vi "Lichen Analysis2.vi"(0 "Parameters (Rejilla)":T2(array[cluster])=[{"Name"="Rectangle 1", "Type"=enum."Rotated Rectangle", "Coordinates"=[0, 0, 80, 76, 0], "Colors"=[16711680], "Drawing Mode"=0, "Text"="Your Text", "Results"=[], "Font, Size & Style"={"Desired Font (Application)"=enum."System Font", "[User-specified Font]"={"Font Name"="Tahoma", "Size"=13, "Strikeout?"=FALSE, "Italic?"=FALSE, "Underline?"=FALSE, "Outline?"=FALSE, "Shadow?"=FALSE, "Bold?"=FALSE, "Rotation Angle"=0.0}, "Horizontal Alignment"=0, "Vertical Alignment"=0}, "Image File Path"=path "", "Use Keying Color"=FALSE}, {"Name"="Rectangle 2", "Type"=enum."Rotated Rectangle", "Coordinates"=[81, 0, 161, 76, 0], "Colors"=[16717824], "Drawing Mode"=0, "Text"="Your Text", "Results"=[], "Font, Size & Style"={"Desired Font (Application)"=enum."System Font", "[User-specified Font]"={"Font Name"="Tahoma", "Size"=13, "Strikeout?"=FALSE, "Italic?"=FALSE, "Underline?"=FALSE, "Outline?"=FALSE, "Shadow?"=FALSE, "Bold?"=FALSE, "Rotation Angle"=0.0}, "Horizontal Alignment"=0, "Vertical Alignment"=0}, "Image File Path"=path "", "Use Keying Color"=FALSE}, {"Name"="Rectangle 3", "Type"=enum."Rotated Rectangle", "Coordinates"=[0, 77, 80, 152, 0], "Colors"=[16717824], "Drawing Mode"=0, "Text"="Your Text", "Results"=[], "Font, Size & Style"={"Desired Font (Application)"=enum."System Font", "[User-specified Font]"={"Font Name"="Tahoma", "Size"=13, "Strikeout?"=FALSE, "Italic?"=FALSE, "Underline?"=FALSE, "Outline?"=FALSE, "Shadow?"=FALSE, "Bold?"=FALSE, "Rotation Angle"=0.0}, "Horizontal Alignment"=0, "Vertical Alignment"=0}, "Image File Path"=path "", "Use Keying Color"=FALSE}, {"Name"="Rectangle 4", "Type"=enum."Rotated Rectangle", "Coordinates"=[81, 77, 161, 152, 0], "Colors"=[16717824], "Drawing Mode"=0, "Text"="Your Text", "Results"=[], "Font, Size & Style"={"Desired Font (Application)"=enum."System Font", "[User-specified Font]"={"Font Name"="Tahoma", "Size"=13, "Strikeout?"=FALSE, "Italic?"=FALSE, "Underline?"=FALSE, "Outline?"=FALSE, "Shadow?"=FALSE, "Bold?"=FALSE, "Rotation Angle"=0.0}, "Horizontal Alignment"=0, "Vertical Alignment"=0}, "Image File Path"=path "", "Use Keying Color"=FALSE}, {"Name"="Rectangle 5", "Type"=enum."Rotated Rectangle", "Coordinates"=[0, 153, 80, 228, 0], "Colors"=[16717824], "Drawing Mode"=0, "Text"="Your Text", "Results"=[], "Font, Size & Style"={"Desired Font (Application)"=enum."System Font", "[User-specified Font]"={"Font Name"="Tahoma", "Size"=13, "Strikeout?"=FALSE, "Italic?"=FALSE, "Underline?"=FALSE, "Outline?"=FALSE, "Shadow?"=FALSE, "Bold?"=FALSE, "Rotation Angle"=0.0}, "Horizontal Alignment"=0, "Vertical Alignment"=0}, "Image File Path"=path "", "Use Keying Color"=FALSE}, {"Name"="Rectangle 6", "Type"=enum."Rotated Rectangle", "Coordinates"=[81, 153, 161, 228, 0], "Colors"=[16717824], "Drawing Mode"=0, "Text"="Your Text", "Results"=[], "Font, Size & Style"={"Desired Font (Application)"=enum."System Font", "[User-specified Font]"={"Font Name"="Tahoma", "Size"=13, "Strikeout?"=FALSE, "Italic?"=FALSE, "Underline?"=FALSE, "Outline?"=FALSE, "Shadow?"=FALSE, "Bold?"=FALSE, "Rotation Angle"=0.0}, "Horizontal Alignment"=0, "Vertical Alignment"=0}, "Image File Path"=path "", "Use Keying Color"=FALSE}, {"Name"="Text 1", "Type"=enum."Text", "Coordinates"=[3, 73], "Colors"=[2817810, 16777216], "Drawing Mode"=0, "Text"="Cell 1", "Results"=[], "Font, Size & Style"={"Desired Font (Application)"=enum."System Font", "[User-specified Font]"={"Font Name"="Tahoma", "Size"=13, "Strikeout?"=FALSE, "Italic?"=FALSE, "Underline?"=FALSE, "Outline?"=FALSE, "Shadow?"=FALSE, "Bold?"=FALSE, "Rotation Angle"=0.0}, "Horizontal Alignment"=0, "Vertical Alignment"=0}, "Image File Path"=path "", "Use Keying Color"=FALSE}, {"Name"="Text 2", "Type"=enum."Text", "Coordinates"=[83, 73], "Colors"=[2817810, 16777216], "Drawing Mode"=0, "Text"="Cell 2", "Results"=[], "Font, Size & Style"={"Desired Font (Application)"=enum."System Font", "[User-specified Font]"={"Font Name"="Tahoma", "Size"=13, "Strikeout?"=FALSE, "Italic?"=FALSE, "Underline?"=FALSE, "Outline?"=FALSE, "Shadow?"=FALSE, "Bold?"=FALSE, "Rotation Angle"=0.0}, "Horizontal Alignment"=0, "Vertical Alignment"=0}, "Image File Path"=path "", "Use Keying Color"=FALSE}, {"Name"="Text 3", "Type"=enum."Text", "Coordinates"=[3, 149], "Colors"=[2817810, 16777216], "Drawing Mode"=0, "Text"="Cell 3", "Results"=[], "Font, Size & Style"={"Desired Font (Application)"=enum."System Font", "[User-specified Font]"={"Font Name"="Tahoma", "Size"=13, "Strikeout?"=FALSE, "Italic?"=FALSE, "Underline?"=FALSE, "Outline?"=FALSE, "Shadow?"=FALSE, "Bold?"=FALSE, "Rotation Angle"=0.0}, "Horizontal Alignment"=0, "Vertical Alignment"=0}, "Image File Path"=path "", "Use Keying Color"=FALSE}, {"Name"="Text 4", "Type"=enum."Text", "Coordinates"=[83, 149], "Colors"=[2817810, 16777216], "Drawing Mode"=0, "Text"="Cell 4", "Results"=[], "Font, Size & Style"={"Desired Font (Application)"=enum."System Font", "[User-specified Font]"={"Font Name"="Tahoma", "Size"=13, "Strikeout?"=FALSE, "Italic?"=FALSE, "Underline?"=FALSE, "Outline?"=FALSE, "Shadow?"=FALSE, "Bold?"=FALSE, "Rotation Angle"=0.0}, "Horizontal Alignment"=0, "Vertical Alignment"=0}, "Image File Path"=path "", "Use Keying Color"=FALSE}, {"Name"="Text 5", "Type"=enum."Text", "Coordinates"=[3, 225], "Colors"=[2817810, 16777216], "Drawing Mode"=0, "Text"="Cell 5", "Results"=[], "Font, Size & Style"={"Desired Font (Application)"=enum."System Font", "[User-specified Font]"={"Font Name"="Tahoma", "Size"=13, "Strikeout?"=FALSE, "Italic?"=FALSE, "Underline?"=FALSE, "Outline?"=FALSE, "Shadow?"=FALSE, "Bold?"=FALSE, "Rotation Angle"=0.0}, "Horizontal Alignment"=0, "Vertical Alignment"=0}, "Image File Path"=path "", "Use Keying Color"=FALSE}, {"Name"="Text 6", "Type"=enum."Text", "Coordinates"=[83, 225], "Colors"=[65407, 16777216], "Drawing Mode"=0, "Text"="Cell 6", "Results"=[], "Font, Size & Style"={"Desired Font (Application)"=enum."System Font", "[User-specified Font]"={"Font Name"="Tahoma", "Size"=13, "Strikeout?"=FALSE, "Italic?"=FALSE, "Underline?"=FALSE, "Outline?"=FALSE, "Shadow?"=FALSE, "Bold?"=FALSE, "Rotation Angle"=0.0}, "Horizontal Alignment"=0, "Vertical Alignment"=0}, "Image File Path"=path "", "Use Keying Color"=FALSE}] {"Colors" format="%.0x"; "Drawing Mode" items=["Frame", "Fill", "Highlight"]; "Results"."String Format" items=["Decimal", "Hexadecimal", "Octal", "Fractional", "Exponential", "Engineering"]; "Font, Size & Style"."Horizontal Alignment" items=["Left", "Center", "Right"]; "Font, Size & Style"."Vertical Alignment" items=["Bottom", "Top", "Baseline"]}, 7 "error in":errorcluster) -> ()   [LabVIEW 2018]
uses:
  <vilib>/vision/NI_Vision_Development_Module.lvlib
panel:
  in  "StationId":u32=1
  out "Array 2":bool[][](array[boolean])
  out "Array":bool[](array[boolean])
  in  "Rows (Default: 3)":i32=3
  in  "Cols (Default: 2)":i32=2
  out "Lichens":T1[](array[plugin-control])
  out "Pixeles":i32[](array[numeric])
  out "?":sgl[](array[numeric])
  out "Original":T1(plugin-control)
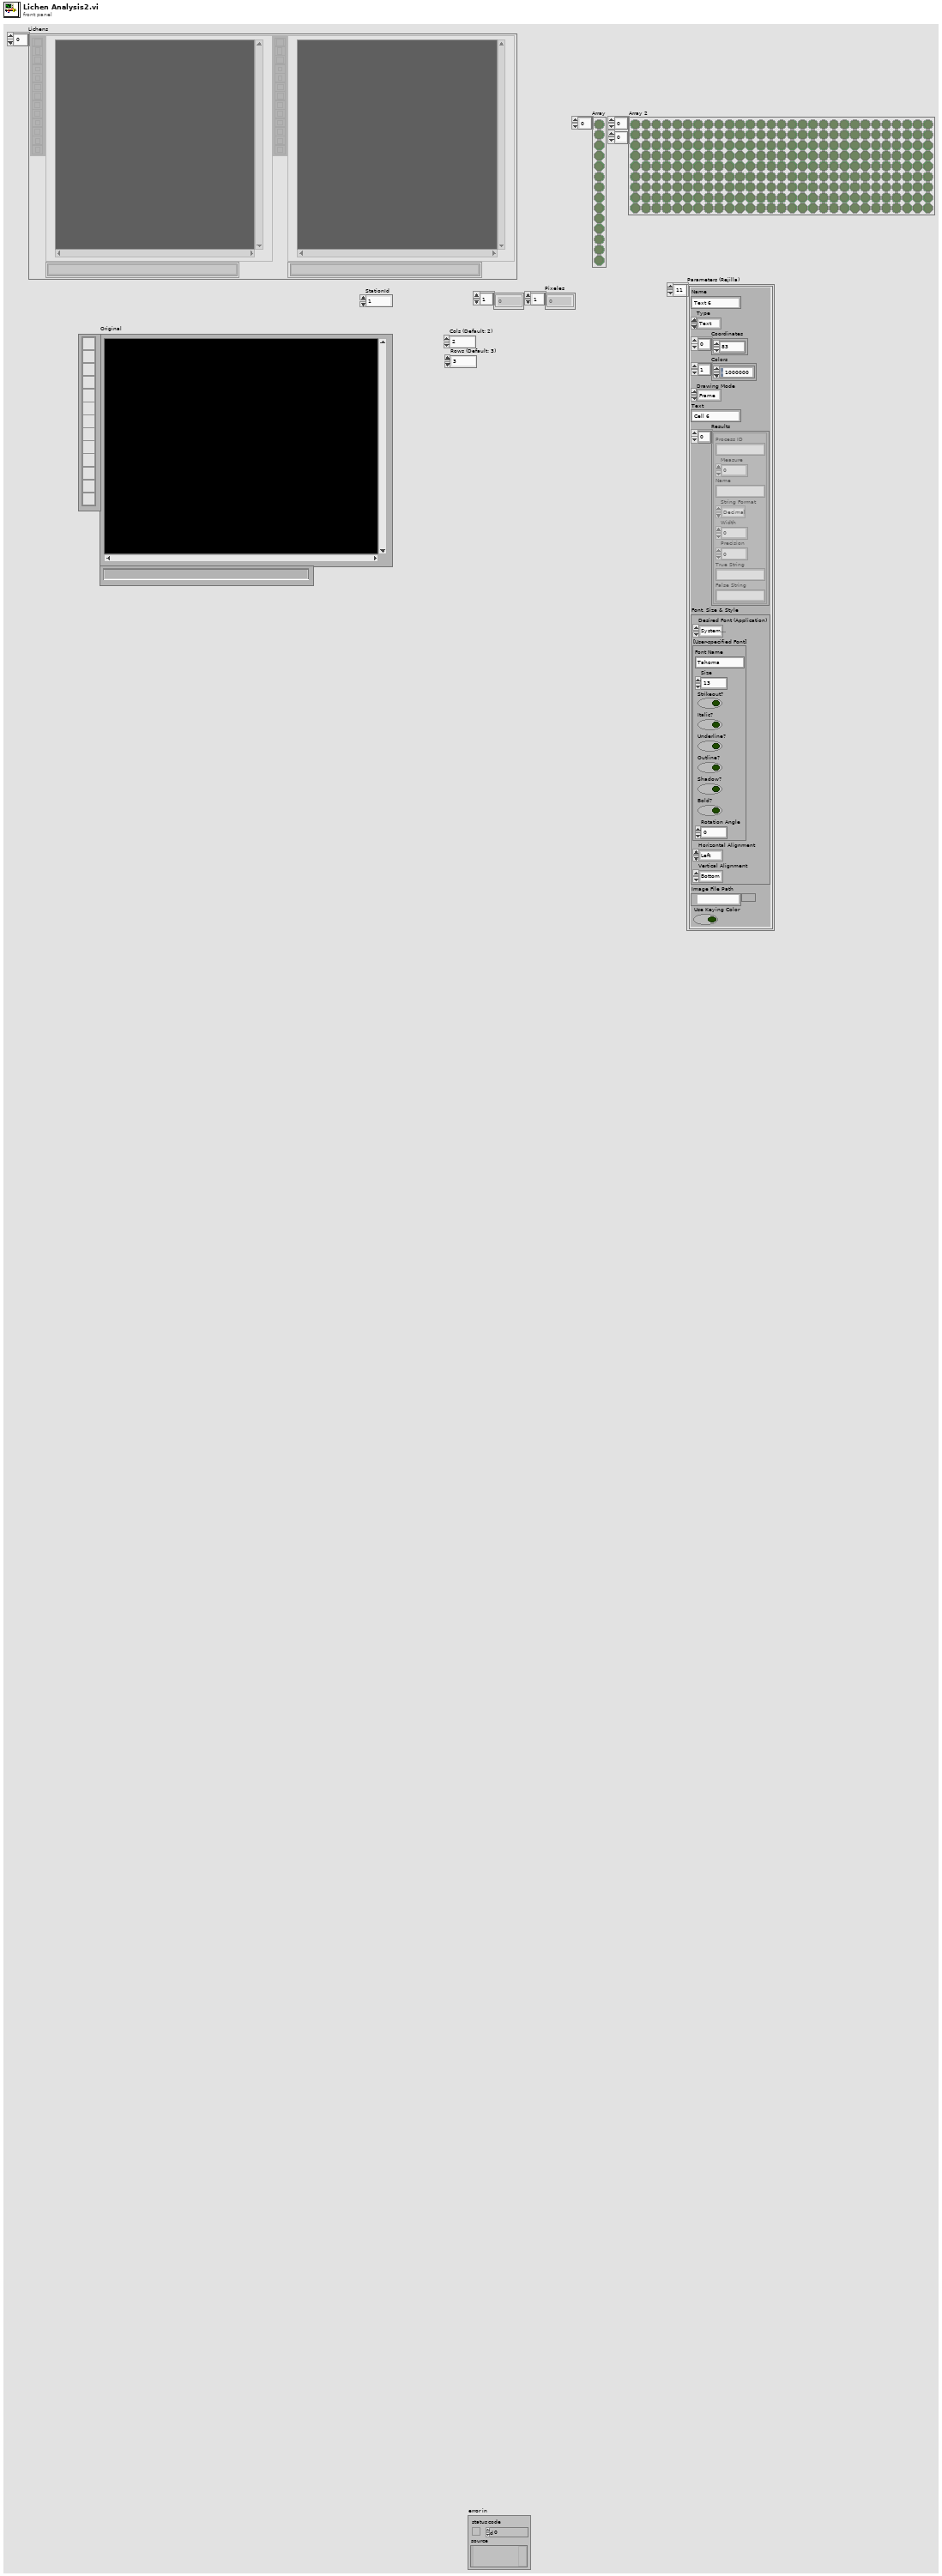
[diagram p1: front panel]
types:
  T1 = typedef "IMAQ Image.ctl" = refnum<image>
  T2 = cluster{"Name":string, "Type":enum16{"Line", "Broken Line", "Free Hand Line", "Rotated Rectangle", "Oval", "Polygon", "Free Hand", "Bitmap", "Text"}, "Coordinates":i32[], "Colors":u32[], "Drawing Mode":u32, "Text":string, "Results":cluster{"Process ID":string, "Measure":u16, "Name":string, "String Format":u16, "Width":i16, "Precision":i16, "True String":string, "False String":string}[], "Font, Size & Style":cluster{"Desired Font (Application)":enum16{"User-specified Font", "Application Font", "System Font", "Dialog Font"}, "[User-specified Font]":cluster{"Font Name":string, "Size":i16, "Strikeout?":bool, "Italic?":bool, "Underline?":bool, "Outline?":bool, "Shadow?":bool, "Bold?":bool, "Rotation Angle":dbl}, "Horizontal Alignment":i16, "Vertical Alignment":i16}, "Image File Path":path, "Use Keying Color":bool}[]
  T3 = typedef "Image Type" = u32
  T4 = cluster{"Position":cluster{"x":sgl, "y":sgl}, "Angle":sgl, "Scale":sgl, "Score":sgl, "Bounding Box":cluster{"x":sgl, "y":sgl}[]}[]
  T5 = cluster{"histogram":u32[], "Minimal Value":sgl, "Maximal Value":sgl, "Starting Value":sgl, "Interval Width":sgl, "Mean Value":sgl, "Standard  Variation":sgl, "Area (pixels)":i32}
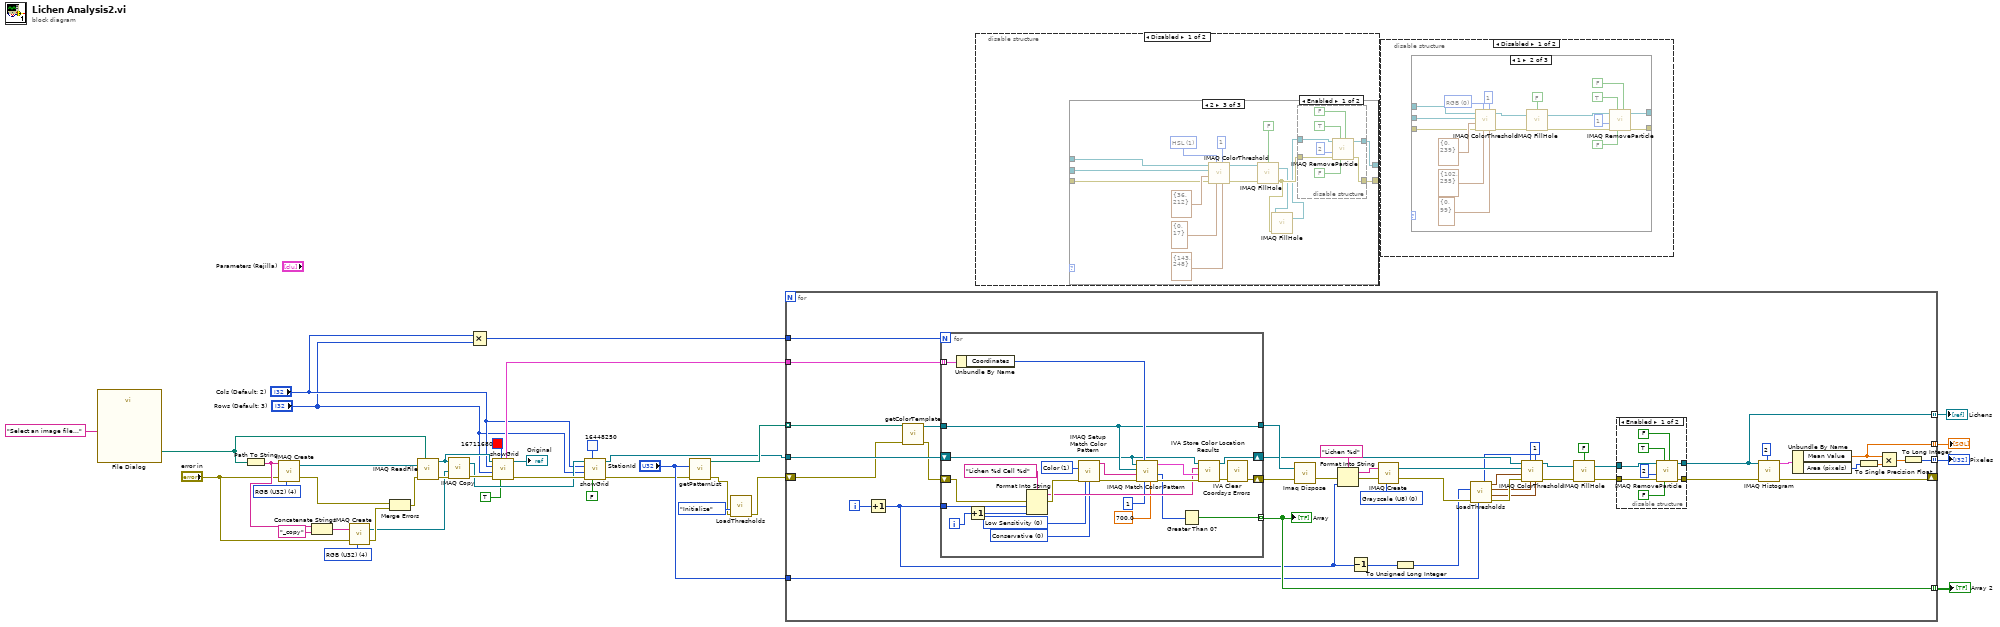
[diagram p0: block diagram]
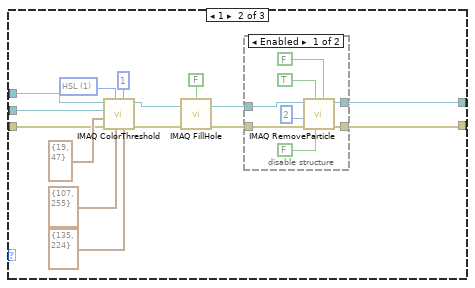
[diagram p3: hidden frame]
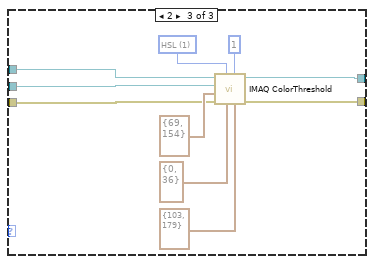
[diagram p8: hidden frame]
diagram:
  w14 = T3 4 items=["Grayscale (U8)", "Grayscale (I16)", "Grayscale (SGL)", "Complex (CSG)", "RGB (U32)", "HSL (U32)", "RGB (U64)", "Grayscale (U16)"] ("Image Type")
  w37 = T3 4 items=["Grayscale (U8)", "Grayscale (I16)", "Grayscale (SGL)", "Complex (CSG)", "RGB (U32)", "HSL (U32)", "RGB (U64)", "Grayscale (U16)"] ("Image Type")
  n1 = call "File Dialog"("prompt"="Select an image file...") -> ("selected path"=w35:path)  [unwired: 6 in, 8 out]
  n2 = Path To String(path=w35) -> (string=w20:string)
  n3 = call "IMAQ Create"("Image Name"=w20, "Image Type"=w37, "error in (no error)"="error in") -> ("New Image"=w36:T1, "error out"=w15:errorcluster)  [unwired: 1 in, 1 out]
  n4 = Concatenate Strings(w20, "_copy" ("string")) -> (w18:string)
  n5 = call "IMAQ Create"("Image Name"=w18, "Image Type"=w14, "error in (no error)"="error in") -> ("New Image"=w12:T1, "error out"=w16:errorcluster)  [unwired: 1 in, 1 out]
  n6 = Merge Errors(w15, w16) -> (w13:errorcluster)
  n7 = call "IMAQ ReadFile"("File Path"=w35, "error in (no error)"=w13, "Image"=w36) -> ("error out"=w22:errorcluster, "Image Out"=w11:T1)  [unwired: 2 in, 5 out]
  n8 = call "IMAQ Copy"("error in (no error)"=w22, "Image Dst"=w12, "Image Src"=w11) -> ("error out"=w21:errorcluster, "Image Dst Out"=w8:T1)  [unwired: 3 in]
  n9 = Multiply(x="Cols (Default: 2)", y="Rows (Default: 3)") -> (x*y=w27:i32)
  n10 = call "showGrid.vi"("Append Text? (True)"=TRUE, "Color (Red)"=u32 16711680, "error in (no error)"=w21, "Rows (Default: 3)"="Rows (Default: 3)", "Cols (Default: 2)"="Cols (Default: 2)", "Image"=w11) -> ("error out"=w10:errorcluster, "Original"=→"Original":T1, "ROIs"=w30:T2)  [unwired: 3 in]
  n11 = call "showGrid.vi"("Append Text? (True)"=FALSE, "Color (Red)"=u32 16448250, "error in (no error)"=w10, "Rows (Default: 3)"="Rows (Default: 3)", "Cols (Default: 2)"="Cols (Default: 2)", "Image"=w8) -> ("error out"=w9:errorcluster, "Original"=w7:T1)  [unwired: 3 in, 1 out]
  n12 = call "getPatternList.vi"("error in"=w9, "StationId"="StationId") -> ("error out"=w24:errorcluster, "TemplatePaths"=w28:path[])  [unwired: 8 in]
  n13 = call "LoadThresholds.vi"("error in"=w24, "Action (Get)"=enum16{"Initialize", "Get"}."Initialize") -> ("error out"=w23:errorcluster)  [unwired: 5 in, 4 out]
  n14 = for {
    tunnel: w7 -> [w81]
    tunnel: w30 -> [w80]
    tunnel: w28 -> [w79] mode=indexing
    shift-right: [w67] -> _
    shift-left: w23 -> [w75]
    tunnel: [w65] -> w34 mode=indexing
    tunnel: [w66] -> w33 mode=indexing
    tunnel: [w58] -> w32 mode=indexing
    tunnel: [w59] -> w29 mode=indexing
    tunnel: w27 -> [w57]
    tunnel: "StationId" -> [w42]
    i -> [w78]
    w72 = T3 0 items=["Grayscale (U8)", "Grayscale (I16)", "Grayscale (SGL)", "Complex (CSG)", "RGB (U32)", "HSL (U32)", "RGB (U64)", "Grayscale (U16)"] ("Image Type")
    n15 = Increment(x=w78) -> (x+1=w40:i32)
    n16 = call "getColorTemplate.vi"("error in (no error)"=w75, "Template Path"=w79) -> ("error out"=w74:errorcluster, "Image Out"=w82:T1)  [unwired: 8 in]
    n17 = for {
      N: w57 -> [_]
      tunnel: w40 -> [w112]
      shift-right: [w102] -> w77
      shift-left: w74 -> [w96]
      tunnel: w82 -> [w95]
      tunnel: w80 -> [w101] mode=indexing
      tunnel: [w98] -> w59 mode=indexing
      shift-right: [w97] -> w50
      shift-left: w81 -> [w94]
      tunnel: [w95] -> w76
      i -> [w93]
      w107 = u32 0 items=["Conservative", "Balance", "Aggressive", "Very Aggressive"] ("Search Strategy")
      w108 = u32 0 items=["Low Sensitivity", "Medium Sensitivity", "High Sensitivity"] ("Color Sensitivity")
      w109 = u32 1 items=["Color and Shape", "Color", "Shape"] ("Match Feature Mode")
      n18 = Unbundle By Name(w101) -> ("Coordinates"=w100:i32[])
      n19 = Increment(x=w93) -> (x+1=w92:i32)
      n20 = Format Into String(format string="Lichen %d Cell %d", error in=w96, w112, w92) -> (resulting string=w110:string, error out=w111:errorcluster)  [unwired: 1 in]
      n21 = call "IMAQ Setup Match Color Pattern"("Match Feature Mode"=w109, "error in (no error)"=w111, "Color Sensitivity"=w108, "Search Strategy"=w107) -> ("Match Color Pattern Setup Data"=w99:string, "error out"=w116:errorcluster)  [unwired: 5 in, 5 out]
      n22 = call "IMAQ Match Color Pattern"("Minimum Match Score"=sgl 700.0, "Number of Matches Requested"=1, "Optional Rectangle"=w100, "error in (no error)"=w116, "Match Color Pattern Setup Data"=w99, "Template Image"=w95, "Image"=w94) -> ("error out"=w115:errorcluster, "Number of Matches"=w104:i32, "Matches"=w114:T4)  [unwired: 2 out]
      n23 = Greater Than 0?(x=w104) -> (x > 0?=w98:bool)
      n24 = call <vilib>:"IVA Store Color Location Results.vi"("error in (no error)"=w115, "Matches"=w114, "Step Name"=w110, "Image in"=w94) -> ("error out"=w103:errorcluster, "Image dup"=w97:T1)  [unwired: 6 out]
      n25 = call <vilib>:"IVA Clear Coordsys Errors.vi"("error in (no error)"=w103) -> ("error out"=w102:errorcluster)  [unwired: 10 in]
    }
    "Array" <- w59
    n26 = call "Imaq Dispose"("Image"=w76, "error in (no error)"=w77) -> ("error out"=w69:errorcluster)  [unwired: 1 in, 3 out]
    n27 = Format Into String(format string="Lichen %d", error in=w69, w40) -> (resulting string=w71:string, error out=w70:errorcluster)  [unwired: 1 in]
    n28 = Decrement(x=w40) -> (x-1=w39:i32)
    n29 = call "IMAQ Create"("Image Name"=w71, "Image Type"=w72, "error in (no error)"=w70) -> ("New Image"=w49:T1, "error out"=w48:errorcluster)  [unwired: 1 in, 1 out]
    n30 = To Unsigned Long Integer(number=w39) -> (unsigned 32bit integer=w41:u32)
    n31 = call "LoadThresholds.vi"("StationId"=w42, "error in"=w48, "Index"=w41) -> ("error out"=w45:errorcluster, "Blue or Luma or Val or Inten Range"=w43:cluster{"Lower value":i32, "Upper value":i32}, "Green or Sat Range"=w44:cluster{"Lower value":i32, "Upper value":i32}, "Red or Hue Range"=w46:cluster{"Lower value":i32, "Upper value":i32}, "Color Mode"=w47:u16)  [unwired: 4 in]
    n32 = call "IMAQ ColorThreshold"("Blue or Luma or Val or Inten Range"=w43, "Replace Value"=1, "Green or Sat Range"=w44, "Color Mode"=w47, "error in (no error)"=w45, "Red or Hue Range"=w46, "Image Dst"=w49, "Image Src"=w50) -> ("error out"=w55:errorcluster, "Image Dst Out"=w54:T1)  [unwired: 2 out]
    n33 = call "IMAQ FillHole"("error in (no error)"=w55, "Image Src"=w54, "Connectivity 4/8 (8)"=FALSE) -> ("error out"=w52:errorcluster, "Image Dst Out"=w51:T1)  [unwired: 1 in, 2 out]
    n34 = disable-structure shown="Enabled" {
      disable-tunnel: [w90 _] -> w68
      disable-tunnel: [w89 w91] -> w58
      disable-tunnel: w52 -> [w84 _]
      disable-tunnel: w51 -> [w83 w91]
      frame Enabled {
        n35 = call "IMAQ RemoveParticle"("Connectivity 4/8 (8)"=FALSE, "Low Pass/High Pass (Low)"=FALSE, "Square/Hexa (Square)"=TRUE, "error in (no error)"=w84, "Number of Erosion"=2, "Image Src"=w83) -> ("error out"=w90:errorcluster, "Image Dst Out"=w89:T1)  [unwired: 4 in]
      }
      frame Disabled {
      }
    }
    n36 = call "IMAQ Histogram"("Number of Classes"=2, "error in (no error)"=w68, "Image"=w58) -> ("error out"=w67:errorcluster, "Histogram Report"=w63:T5)  [unwired: 2 in, 5 out]
    n37 = Unbundle By Name(w63) -> ("Mean Value"=w65:sgl, "Area (pixels)"=w61:i32)
    n38 = To Single Precision Float(number=w61) -> (single precision float=w60:sgl)
    n39 = Multiply(x=w65, y=w60) -> (x*y=w62:sgl)
    n40 = To Long Integer(number=w62) -> (32bit integer=w66:i32)
  }
  "?" <- w34
  "Pixeles" <- w33
  "Lichens" <- w32
  "Array 2" <- w29
  n41 = disable-structure shown="Disabled" {
    frame Disabled {
      n42 = case shown="2" {
        selector: _ -> [_ _ _]
        tunnel: _ -> [w118 w128 w152]
        tunnel: _ -> [w117 w125 w153]
        tunnel: [w118 w124 w147] -> _
        tunnel: [w117 w123 w146] -> _
        tunnel: _ -> [_ w122 w151]
        frame 0, Default {
        }
        frame 1 {
          w132 = u16 1 items=["RGB", "HSL", "HSV", "HSI"] ("Color Mode")
          n43 = call "IMAQ ColorThreshold"("Blue or Luma or Val or Inten Range"=cluster{"Lower value":i32, "Upper value":i32} {"Lower value"=135, "Upper value"=224}, "Replace Value"=1, "Green or Sat Range"=cluster{"Lower value":i32, "Upper value":i32} {"Lower value"=107, "Upper value"=255}, "Color Mode"=w132, "error in (no error)"=w128, "Red or Hue Range"=cluster{"Lower value":i32, "Upper value":i32} {"Lower value"=19, "Upper value"=47}, "Image Dst"=w122, "Image Src"=w125) -> ("error out"=w127:errorcluster, "Image Dst Out"=w126:T1)  [unwired: 2 out]
          n44 = call "IMAQ FillHole"("error in (no error)"=w127, "Image Src"=w126, "Connectivity 4/8 (8)"=FALSE) -> ("error out"=w120:errorcluster, "Image Dst Out"=w119:T1)  [unwired: 1 in, 2 out]
          n45 = disable-structure shown="Enabled" {
            disable-tunnel: [w141 _] -> w124
            disable-tunnel: [w140 w142] -> w123
            disable-tunnel: w120 -> [w135 _]
            disable-tunnel: w119 -> [w134 w142]
            frame Enabled {
              n46 = call "IMAQ RemoveParticle"("Connectivity 4/8 (8)"=FALSE, "Low Pass/High Pass (Low)"=FALSE, "Square/Hexa (Square)"=TRUE, "error in (no error)"=w135, "Number of Erosion"=2, "Image Src"=w134) -> ("error out"=w141:errorcluster, "Image Dst Out"=w140:T1)  [unwired: 4 in]
            }
            frame Disabled {
            }
          }
        }
        frame 2 {
          w157 = u16 1 items=["RGB", "HSL", "HSV", "HSI"] ("Color Mode")
          n47 = call "IMAQ ColorThreshold"("Blue or Luma or Val or Inten Range"=cluster{"Lower value":i32, "Upper value":i32} {"Lower value"=143, "Upper value"=248}, "Replace Value"=1, "Green or Sat Range"=cluster{"Lower value":i32, "Upper value":i32} {"Lower value"=0, "Upper value"=17}, "Color Mode"=w157, "error in (no error)"=w152, "Red or Hue Range"=cluster{"Lower value":i32, "Upper value":i32} {"Lower value"=36, "Upper value"=212}, "Image Dst"=w151, "Image Src"=w153) -> ("error out"=w149:errorcluster, "Image Dst Out"=w148:T1)  [unwired: 2 out]
          n48 = call "IMAQ FillHole"("error in (no error)"=w149, "Image Src"=w148, "Connectivity 4/8 (8)"=FALSE) -> ("error out"=w145:errorcluster, "Image Dst Out"=w144:T1)  [unwired: 1 in, 2 out]
          n49 = call "IMAQ FillHole"("error in (no error)"=w145, "Image Src"=w144) -> ("Image Dst Out"=w143:T1)  [unwired: 2 in, 3 out]
          n50 = disable-structure shown="Enabled" {
            disable-tunnel: w143 -> [w159 w167]
            disable-tunnel: w145 -> [w162 _]
            disable-tunnel: [w161 _] -> w147
            disable-tunnel: [w160 w167] -> w146
            frame Enabled {
              n51 = call "IMAQ RemoveParticle"("Connectivity 4/8 (8)"=FALSE, "Low Pass/High Pass (Low)"=FALSE, "Square/Hexa (Square)"=TRUE, "error in (no error)"=w162, "Number of Erosion"=2, "Image Src"=w159) -> ("error out"=w161:errorcluster, "Image Dst Out"=w160:T1)  [unwired: 1 in, 3 out]
            }
            frame Disabled {
            }
          }
        }
      }
    }
    frame Enabled {
    }
  }
  n52 = disable-structure shown="Disabled" {
    frame Disabled {
      n53 = case shown="1" {
        selector: _ -> [_ _ _]
        tunnel: _ -> [w169 w183 w190]
        tunnel: _ -> [w168 w173 w193]
        tunnel: [w169 w172 w192] -> _
        tunnel: [w168 w171 w191] -> _
        tunnel: _ -> [_ w170 w189]
        frame 0, Default {
        }
        frame 1 {
          w187 = u16 0 items=["RGB", "HSL", "HSV", "HSI"] ("Color Mode")
          n54 = call "IMAQ ColorThreshold"("Blue or Luma or Val or Inten Range"=cluster{"Lower value":i32, "Upper value":i32} {"Lower value"=0, "Upper value"=99}, "Replace Value"=1, "Green or Sat Range"=cluster{"Lower value":i32, "Upper value":i32} {"Lower value"=102, "Upper value"=255}, "Color Mode"=w187, "error in (no error)"=w183, "Red or Hue Range"=cluster{"Lower value":i32, "Upper value":i32} {"Lower value"=0, "Upper value"=239}, "Image Dst"=w170, "Image Src"=w173) -> ("error out"=w177:errorcluster, "Image Dst Out"=w174:T1)  [unwired: 2 out]
          n55 = call "IMAQ FillHole"("error in (no error)"=w177, "Image Src"=w174, "Connectivity 4/8 (8)"=FALSE) -> ("error out"=w176:errorcluster, "Image Dst Out"=w175:T1)  [unwired: 1 in, 2 out]
          n56 = call "IMAQ RemoveParticle"("Connectivity 4/8 (8)"=FALSE, "Low Pass/High Pass (Low)"=FALSE, "Square/Hexa (Square)"=TRUE, "error in (no error)"=w176, "Number of Erosion"=1, "Image Src"=w175) -> ("error out"=w172:errorcluster, "Image Dst Out"=w171:T1)  [unwired: 1 in, 3 out]
        }
        frame 2 {
          w197 = u16 1 items=["RGB", "HSL", "HSV", "HSI"] ("Color Mode")
          n57 = call "IMAQ ColorThreshold"("Blue or Luma or Val or Inten Range"=cluster{"Lower value":i32, "Upper value":i32} {"Lower value"=103, "Upper value"=179}, "Replace Value"=1, "Green or Sat Range"=cluster{"Lower value":i32, "Upper value":i32} {"Lower value"=0, "Upper value"=36}, "Color Mode"=w197, "error in (no error)"=w190, "Red or Hue Range"=cluster{"Lower value":i32, "Upper value":i32} {"Lower value"=69, "Upper value"=154}, "Image Dst"=w189, "Image Src"=w193) -> ("error out"=w192:errorcluster, "Image Dst Out"=w191:T1)  [unwired: 2 out]
        }
      }
    }
    frame Enabled {
    }
  }
